vi "Third-octave Range to Band Number.vi"(1 "frequency range":T1={"low band"=enum."125 Hz", "high band"=enum."8000 Hz"}) -> (0 "band number":cluster{"low band":i32, "high band":i32})   [LabVIEW 2017]
doc: "Converts the selected third-octave frequency range to the corresponding band number.\nThe band number is based on the low and high bands specified in the frequency range cluster. A value of 0 corresponds to the reference frequency of the audio-frequency range, 1 kHz. Each successive value corresponds to the next third-octave band. Positive values cover the range above 1 kHz, and negative values cover the range below 1 kHz.\nThe frequency range cluster uses a pre-defined list of frequencies from 20 Hz to 20 kHz in third-octave steps. If you need to use any other specific frequency outside of this frequency range, you should use the Frequency Range to Band Number VI instead."
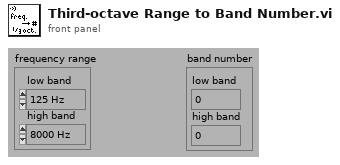
[diagram p1: front panel]
types:
  T1 = cluster{"low band":enum16{"20 Hz", "25 Hz", "31.5 Hz", "40 Hz", "50 Hz", "63 Hz", "80 Hz", "100 Hz", "125 Hz", "160 Hz", "200 Hz", "250 Hz", "315 Hz", "400 Hz", "500 Hz", "630 Hz", "800 Hz", "1000 Hz", "1250 Hz", "1600 Hz", "2000 Hz", "2500 Hz", "3150 Hz", "4000 Hz", "5000 Hz", "6300 Hz", "8000 Hz", "10000 Hz", "12500 Hz", "16000 Hz", "20000 Hz"}, "high band":enum16{"20 Hz", "25 Hz", "31.5 Hz", "40 Hz", "50 Hz", "63 Hz", "80 Hz", "100 Hz", "125 Hz", "160 Hz", "200 Hz", "250 Hz", "315 Hz", "400 Hz", "500 Hz", "630 Hz", "800 Hz", "1000 Hz", "1250 Hz", "1600 Hz", "2000 Hz", "2500 Hz", "3150 Hz", "4000 Hz", "5000 Hz", "6300 Hz", "8000 Hz", "10000 Hz", "12500 Hz", "16000 Hz", "20000 Hz"}}
  T2 = enum16{"20 Hz", "25 Hz", "31.5 Hz", "40 Hz", "50 Hz", "63 Hz", "80 Hz", "100 Hz", "125 Hz", "160 Hz", "200 Hz", "250 Hz", "315 Hz", "400 Hz", "500 Hz", "630 Hz", "800 Hz", "1000 Hz", "1250 Hz", "1600 Hz", "2000 Hz", "2500 Hz", "3150 Hz", "4000 Hz", "5000 Hz", "6300 Hz", "8000 Hz", "10000 Hz", "12500 Hz", "16000 Hz", "20000 Hz"}
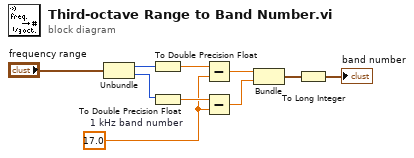
[diagram p0: block diagram]
diagram:
  w5 = 17.0  # 1 kHz band number
  n1 = Unbundle("frequency range") -> ("low band"=w9:T2, "high band"=w10:T2)
  n2 = To Double Precision Float(number=w9) -> (double precision float=w7:dbl)
  n3 = To Double Precision Float(number=w10) -> (double precision float=w8:dbl)
  n4 = Subtract(x=w7, y=w5) -> (x-y=w2:dbl)
  n5 = Subtract(x=w8, y=w5) -> (x-y=w1:dbl)
  n6 = Bundle(w2, w1) -> (w4:cluster{dbl, dbl})  [unwired: 1 in]
  n7 = To Long Integer(number=w4) -> (32bit integer=→"band number":cluster{i32, i32})
